vi "Constant Move Speed Test.vi"   [LabVIEW 2015]
panel:
  # "1 is the dumping position"
  # "Auto = true\nMaunal = false"
  # "zero is level"
  # "Reverse"
  # "Forward"
  # "Up"
  # "Down"
  # "CW"
  # "CCW"
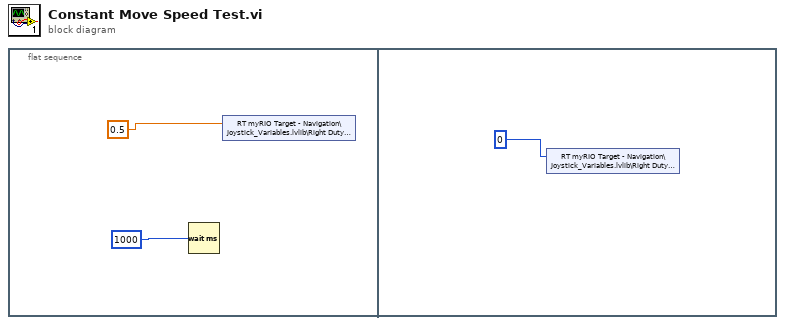
[diagram p0: block diagram]
diagram:
  n1 = flat-sequence {
    frame #0 {
      n2 = Wait (ms)(milliseconds to wait=1000) -> ()  [unwired: 1 out]
      n3 = shared-variable "RT myRIO Target - Navigation\\Joystick_Variables.lvlib\\Right Duty Cycle"(0.5) -> ()  [unwired: 1 in, 1 out]
    }
    frame #1 {
      n4 = shared-variable "RT myRIO Target - Navigation\\Joystick_Variables.lvlib\\Right Duty Cycle"(0) -> ()  [unwired: 1 in, 1 out]
    }
  }
